vi "Create_directory_path.vi"(1 "Path name":path) -> (0 "Path name Out":path)   [LabVIEW 2010]
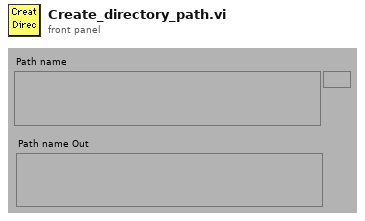
[diagram p1: front panel]
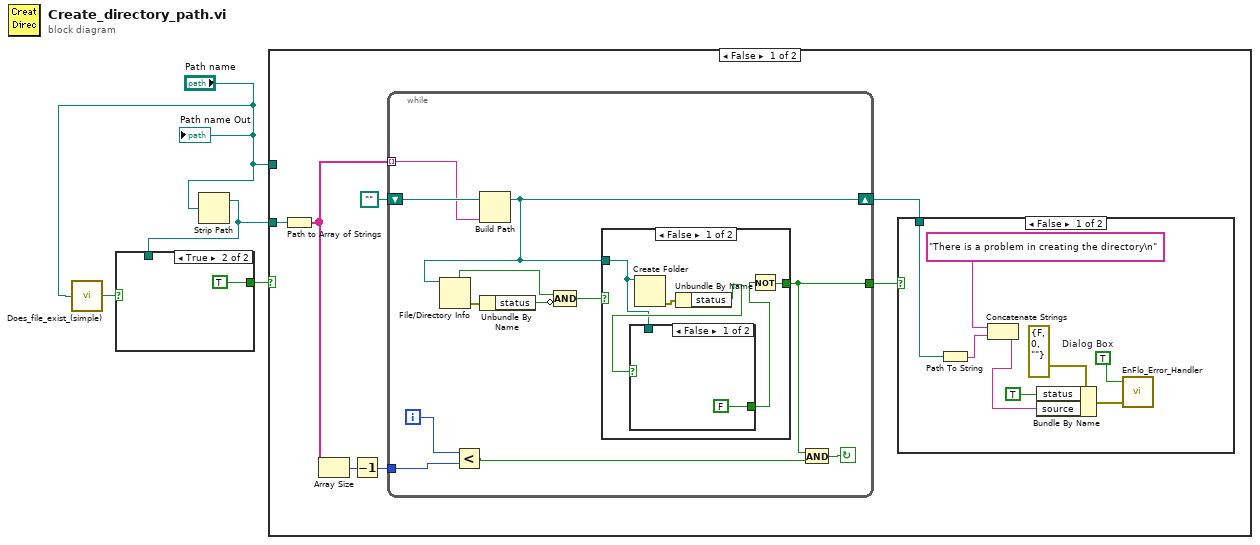
[diagram p0: block diagram]
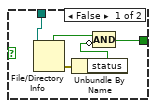
[diagram p2: hidden frame]
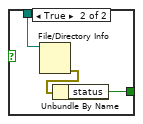
[diagram p3: hidden frame]
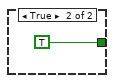
[diagram p4: hidden frame]
diagram:
  n1 = call "Does_file_exist_(simple).vi"("Pathname"="Path name") -> ("exists?"=w2:bool)
  n2 = Strip Path(path="Path name") -> (stripped path=w3:path)  [unwired: 1 out]
  n3 = case shown="True" w2 {
    tunnel: [w8 TRUE] -> w4
    tunnel: w3 -> [w5 _]
    frame False {
      n4 = File/Directory Info(path=w5) -> (directory=w6:bool, error out=w9:errorcluster)  [unwired: 1 in, 5 out]
      n5 = Unbundle By Name(w9) -> ("status"=w7:bool)
      n6 = Compound Arithmetic op=AND(w6, invert w7) -> (w8:bool)
    }
    frame True {
    }
  }
  n7 = case shown="False" w4 {
    tunnel: "Path name" -> [_ _]
    tunnel: w3 -> [w12 _]
    frame False {
      n8 = Path to Array of Strings(0:w12) -> (2:w16:string[])  [unwired: 1 out]
      n9 = Array Size(array=w16) -> (size(s)=w11:i32)
      n10 = Decrement(x=w11) -> (x-1=w13:i32)
      n11 = while {
        tunnel: [w23] -> w15
        tunnel: w13 -> [w26]
        shift-left: path "" ("appended path") -> [w29]
        shift-right: [w22] -> w14
        tunnel: w16 -> [w28] mode=indexing
        i -> [w27]
        stop <- w24 continue-if-true
        n12 = Less?(x=w27, y=w26) -> (x < y?=w25:bool)
        n13 = Build Path(base path=w29, name or relative path=w28) -> (appended path=w22:path)
        n14 = File/Directory Info(path=w22) -> (directory=w19:bool, error out=w21:errorcluster)  [unwired: 1 in, 5 out]
        n15 = Unbundle By Name(w21) -> ("status"=w20:bool)
        n16 = Compound Arithmetic op=AND(w19, invert w20) -> (w18:bool)
        n17 = case shown="False" w18 {
          tunnel: w22 -> [w31 _]
          tunnel: [w33 TRUE] -> w23
          frame False {
            n18 = Create Folder(path (use dialog)=w31) -> (error out=w34:errorcluster)  [unwired: 1 in, 3 out]
            n19 = Unbundle By Name(w34) -> ("status"=w32:bool)
            n20 = case shown="False" w32 {
              tunnel: w31 -> [_ w38]
              tunnel: [FALSE ("status") w36] -> w30
              frame False {
              }
              frame True {
                n21 = File/Directory Info(path=w38) -> (error out=w37:errorcluster)  [unwired: 1 in, 6 out]
                n22 = Unbundle By Name(w37) -> ("status"=w36:bool)
              }
            }
            n23 = Not(x=w30) -> (.not. x?=w33:bool)
          }
          frame True {
          }
        }
        n24 = And(x=w23, y=w25) -> (x .and. y?=w24:bool)
      }
      n25 = case shown="False" w15 {
        tunnel: w14 -> [w47 _]
        frame False {
          w42 = TRUE  # Dialog Box
          n26 = Path To String(path=w47) -> (string=w45:string)
          n27 = Concatenate Strings("There is a problem in creating the directory\n", w45) -> (w40:string)
          n28 = Bundle By Name(cluster=errorcluster {"status"=FALSE, "code"=0, "source"=""} ("error in (no error)"), "status"=TRUE ("Bundle Element"), "source"=w40) -> (w43:errorcluster)
          n29 = call "EnFlo_Error_Handler.vi"("error in (no error)"=w43, "Dialog Box (T)"=w42) -> ()  [unwired: 1 in, 3 out]
        }
        frame True {
        }
      }
    }
    frame True {
    }
  }
  "Path name Out" <- "Path name"
